vi "1 NanoStructure NS.vi"(6 "m-nm 4":dbl, 9 "Length of Base":dbl, 10 "m-nm WB":dbl, 11 "Width of Base":dbl) -> (1 "NS Width":dbl, 2 "NS Length":dbl, 3 "NS Base Area":dbl)   [LabVIEW 2020]
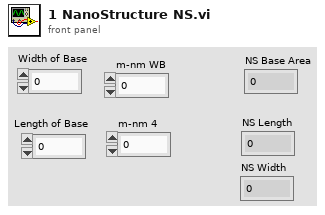
[diagram p1: front panel]
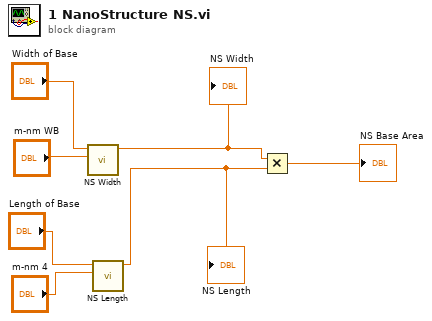
[diagram p0: block diagram]
diagram:
  n1 = call "NS Width.vi"("m-nm WB"="m-nm WB", "Width of Base"="Width of Base") -> ("Numeric"=w5:dbl)  [unwired: 9 in]
  "NS Width" <- w5
  n2 = call "NS Length.vi"("m-nm NS base"="m-nm 4", "Length of Base"="Length of Base") -> ("Numeric"=w6:dbl)  [unwired: 9 in]
  "NS Length" <- w6
  n3 = Multiply(x=w5, y=w6) -> (x*y=→"NS Base Area":dbl)
